vi "cRIO monitor.vi"() -> ()   [LabVIEW 2016]
doc: "This VI is part of the Top Level library of VIs that are run upon startup of Main Control program. cRIO hardware and network connections are monitored."
uses:
  <vilib>/Utility/miscctls.llb/LVRowAndColumnTypeDef.ctl
  Top Level.lvlib
panel:
  in  "Tab Control":enum32{"Network", "Resources", "VI Errors"}(tab)
  out "cRIO network connections":i32(listbox)
  in  "Ping Timeout (ms)":i32=100
  out "cRIO hardware status":i32(listbox)
  in  "Clear SV Error":bool
  out "Ping error":errorcluster
  out "SV read error":errorcluster
  in  "Clear Ping Error":bool
  in  "stop":bool
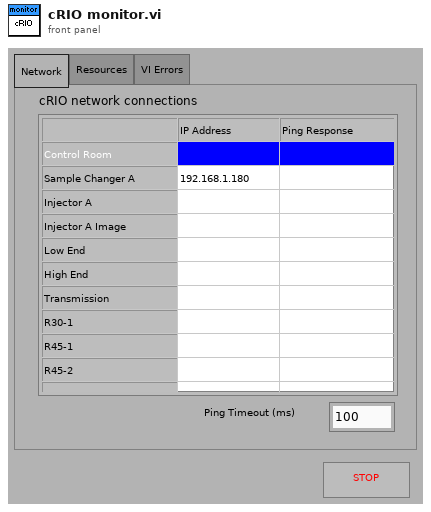
[diagram p1: front panel]
types:
  T1 = typedef "LVRowAndColumnTypeDef.ctl" = cluster{"Row":i32, "Column":i32}
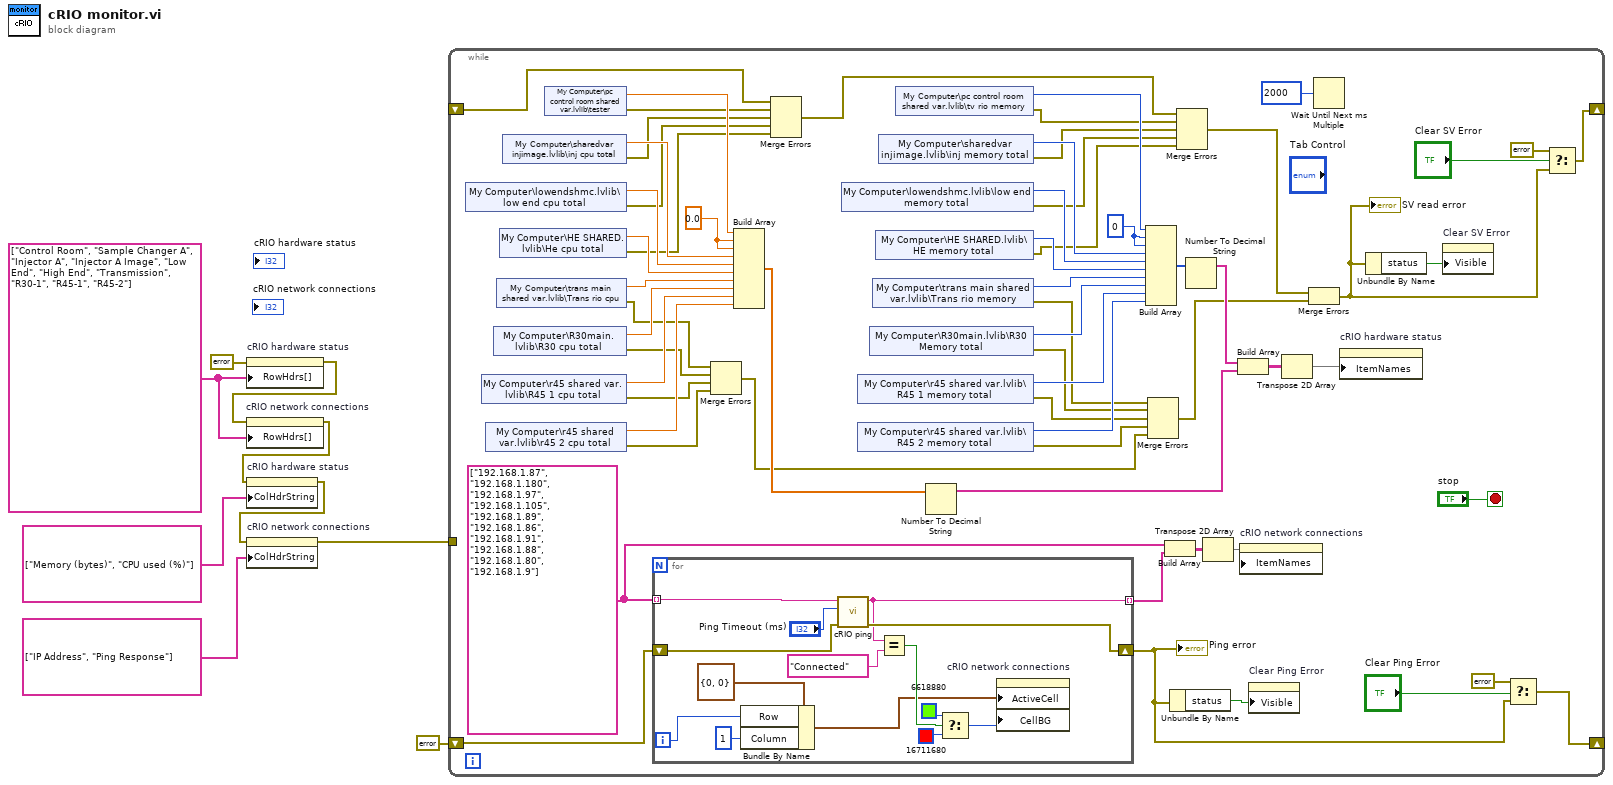
[diagram p0: block diagram]
diagram:
  w9 = string[] ["Control Room", "Sample Changer A", "Injector A", "Injector A Image", "Low End", "High End", "Transmission", "R30-1", "R45-1", "R45-2"]
  n1 = property on="cRIO hardware status" class="MCListbox (strict)"(error in=errorcluster {"status"=FALSE, "code"=0, "source"=""} ("error out"), "RowHdrs[]"=w9) -> (error out=w8:errorcluster)  [unwired: 1 in, 1 out]
  n2 = property on="cRIO network connections" class="MCListbox (strict)"(error in=w8, "RowHdrs[]"=w9) -> (error out=w7:errorcluster)  [unwired: 1 in, 1 out]
  n3 = property on="cRIO hardware status" class="MCListbox (strict)"(error in=w7, "ColHdrString"=string[] ["Memory (bytes)", "CPU used (%)"]) -> (error out=w6:errorcluster)  [unwired: 1 in, 1 out]
  n4 = property on="cRIO network connections" class="MCListbox (strict)"(error in=w6, "ColHdrString"=string[] ["IP Address", "Ping Response"]) -> (error out=w2:errorcluster)  [unwired: 1 in, 1 out]
  n5 = while {
    shift-right: [w11] -> _
    shift-left: _ -> [w36]
    shift-right: [w18] -> _
    shift-left: errorcluster {"status"=FALSE, "code"=0, "source"=""} ("Ping error out") -> [w47]
    tunnel: w2 -> [_]
    stop <- "stop" stop-if-true
    w49 = string[] ["192.168.1.87", "192.168.1.180", "192.168.1.97", "192.168.1.105", "192.168.1.89", "192.168.1.86", "192.168.1.91", "192.168.1.88", "192.168.1.80", "192.168.1.9"]
    w50 = u32 0 ("element")
    w51 = 0.0 ("element")
    n6 = shared-variable "My Computer\\lowendshmc.lvlib\\low end cpu total"() -> (w67:dbl, error out=w38:errorcluster)  [unwired: 1 in]
    n7 = shared-variable "My Computer\\r45 shared var.lvlib\\R45 1 cpu total"() -> (w63:dbl, error out=w35:errorcluster)  [unwired: 1 in]
    n8 = shared-variable "My Computer\\r45 shared var.lvlib\\r45 2 cpu total"() -> (w62:dbl, error out=w32:errorcluster)  [unwired: 1 in]
    n9 = shared-variable "My Computer\\R30main.lvlib\\R30 cpu total"() -> (w64:dbl, error out=w34:errorcluster)  [unwired: 1 in]
    n10 = shared-variable "My Computer\\trans main shared var.lvlib\\Trans rio cpu"() -> (w65:dbl, error out=w33:errorcluster)  [unwired: 1 in]
    n11 = shared-variable "My Computer\\HE SHARED.lvlib\\He cpu total"() -> (w66:dbl, error out=w37:errorcluster)  [unwired: 1 in]
    n12 = shared-variable "My Computer\\sharedvar injimage.lvlib\\inj cpu total"() -> (w68:dbl, error out=w39:errorcluster)  [unwired: 1 in]
    n13 = shared-variable "My Computer\\pc control room shared var.lvlib\\tester"() -> (w69:dbl, error out=w40:errorcluster)  [unwired: 1 in]
    n14 = for {
      tunnel: w49 -> [w84] mode=indexing
      tunnel: [w81] -> w48 mode=indexing
      shift-right: [w82] -> w16
      shift-left: w47 -> [w83]
      i -> [w74]
      n15 = Bundle By Name(cluster=T1 {"Row"=0, "Column"=0} ("Active Cell:Active Cell"), "Row"=w74, "Column"=1) -> (w73:T1)
      n16 = call "cRIO ping.vi"("Error in"=w83, "Ping Timeout (ms)"="Ping Timeout (ms)", "IP Address"=w84) -> ("Ping error out"=w82:errorcluster, "Ping Response"=w81:string)  [unwired: 7 in]
      n17 = Equal?(x=w81, y="Connected" ("t")) -> (x = y?=w78:bool)
      n18 = Select(t=u32 6618880, s=w78, f=u32 16711680) -> (s? t:f=w79:u32)
      n19 = property on="cRIO network connections" class="MCListbox (strict)"("ActiveCell"=w73, "CellBG"=w79) -> ()  [unwired: 2 in, 2 out]
    }
    "Ping error" <- w16
    n20 = Merge Errors(w33, w34, w35, w32) -> (w21:errorcluster)
    n21 = Build Array(w69, w51, w51, w68, w67, w66, w65, w64, w63, w62) -> (w52:dbl[])
    n22 = Merge Errors(w36, w40, w39, w38, w37) -> (w31:errorcluster)
    n23 = shared-variable "My Computer\\lowendshmc.lvlib\\low end memory total"() -> (w55:u32, error out=w28:errorcluster)  [unwired: 1 in]
    n24 = shared-variable "My Computer\\r45 shared var.lvlib\\R45 1 memory total"() -> (w59:u32, error out=w25:errorcluster)  [unwired: 1 in]
    n25 = shared-variable "My Computer\\r45 shared var.lvlib\\R45 2 memory total"() -> (w60:u32, error out=w26:errorcluster)  [unwired: 1 in]
    n26 = shared-variable "My Computer\\R30main.lvlib\\R30 Memory total"() -> (w58:u32, error out=w24:errorcluster)  [unwired: 1 in]
    n27 = shared-variable "My Computer\\trans main shared var.lvlib\\Trans rio memory"() -> (w57:u32, error out=w23:errorcluster)  [unwired: 1 in]
    n28 = shared-variable "My Computer\\HE SHARED.lvlib\\HE memory total"() -> (w54:u32, error out=w27:errorcluster)  [unwired: 1 in]
    n29 = shared-variable "My Computer\\sharedvar injimage.lvlib\\inj memory total"() -> (w56:u32, error out=w29:errorcluster)  [unwired: 1 in]
    n30 = shared-variable "My Computer\\pc control room shared var.lvlib\\tv rio memory"() -> (w61:u32, error out=w30:errorcluster)  [unwired: 1 in]
    n31 = Number To Decimal String(number=w52) -> (decimal integer string=w44:string[])  [unwired: 1 in]
    n32 = Build Array(w61, w50, w50, w56, w55, w54, w57, w58, w59, w60) -> (w53:u32[])
    n33 = Merge Errors(w23, w24, w25, w26, w21) -> (w22:errorcluster)
    n34 = Build Array(w49, w48) -> (w46:string[][])
    n35 = Unbundle By Name(w16) -> ("status"=w19:bool)
    n36 = Merge Errors(w31, w30, w29, w28, w27) -> (w20:errorcluster)
    n37 = Number To Decimal String(number=w53) -> (decimal integer string=w45:string[])  [unwired: 1 in]
    n38 = Transpose 2D Array(2D array=w46) -> (transposed array=w41:string[][])
    n39 = Build Array(w45, w44) -> (w43:string[][])
    n40 = property on="cRIO network connections" class="MCListbox (strict)"("ItemNames"=w41) -> ()  [unwired: 2 in, 2 out]
    n41 = property on="Clear Ping Error" class="Bool"("Visible"=w19) -> ()  [unwired: 2 in, 2 out]
    n42 = Transpose 2D Array(2D array=w43) -> (transposed array=w42:string[][])
    n43 = Merge Errors(w20, w22) -> (w10:errorcluster)
    "SV read error" <- w10
    n44 = Wait Until Next ms Multiple(millisecond multiple=u32 2000) -> ()  [unwired: 1 out]
    n45 = property on="cRIO hardware status" class="MCListbox (strict)"("ItemNames"=w42) -> ()  [unwired: 2 in, 2 out]
    n46 = Unbundle By Name(w10) -> ("status"=w14:bool)
    n47 = property on="Clear SV Error" class="Bool"("Visible"=w14) -> ()  [unwired: 2 in, 2 out]
    n48 = Select(t=errorcluster {"status"=FALSE, "code"=0, "source"=""}, s="Clear Ping Error", f=w16) -> (s? t:f=w18:errorcluster)
    n49 = Select(t=errorcluster {"status"=FALSE, "code"=0, "source"=""}, s="Clear SV Error", f=w10) -> (s? t:f=w11:errorcluster)
  }
